vi "iRobot UART Read Flush.vi"(8 "error in":errorcluster, 11 "UART port in":T1) -> (0 "error out":errorcluster, 1 "data":u8[](array[numeric]), 3 "UART port out":T1)   [LabVIEW 2014]
doc: "Read all available data from the UART receive buffer."
uses:
  iRobot UART Port Type.ctl
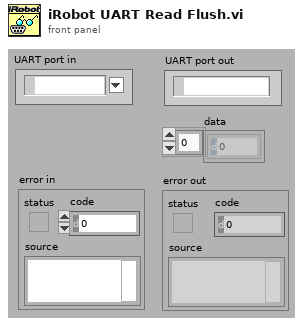
[diagram p1: front panel]
types:
  T1 = typedef "iRobot UART Port Type.ctl" = refnum<visa-resource-name>
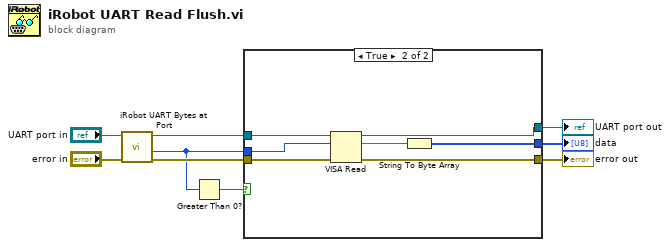
[diagram p0: block diagram]
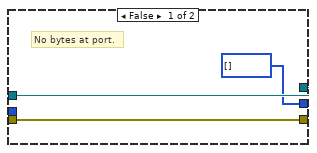
[diagram p2: hidden frame]
diagram:
  n1 = call "iRobot UART Bytes at Port.vi"("error in"="error in", "UART port in"="UART port in") -> ("error out"=w5:errorcluster, "bytes at port"=w4:u32, "UART port out"=w6:T1)  [unwired: 1 in, 6 out]
  n2 = Greater Than 0?(x=w4) -> (x > 0?=w3:bool)
  n3 = case shown="True" w3 {
    tunnel: w6 -> [w11 w19]
    tunnel: w4 -> [_ w18]
    tunnel: w5 -> [w12 w17]
    tunnel: [w12 w14] -> w9
    tunnel: [w11 w16] -> w2
    tunnel: [u8[] [] ("data") w15] -> w1
    frame False {
      # "No bytes at port."
    }
    frame True {
      n4 = VISA Read(VISA resource name=w19, byte count=w18, error in (no error)=w17) -> (VISA resource name out=w16:T1, read buffer=w13:string, error out=w14:errorcluster)  [unwired: 1 out]
      n5 = String To Byte Array(string=w13) -> (unsigned byte array=w15:u8[])
    }
  }
  "data" <- w1
  "UART port out" <- w2
  "error out" <- w9
